vi "9217 4Ch RTD Input.vi"(1 "9217 I/O":T1={"9217 RTD0"="NI 9217/RTD0", "9217 RTD1"="NI 9217/RTD1", "9217 RTD2"="NI 9217/RTD2", "9217 RTD3"="NI 9217/RTD3"}) -> (0 "Packets":u64[](array[numeric]))   [LabVIEW 2010]
uses:
  <vilib>/eio/EIONode/EIONode.xnode
  <vilib>/rvi/eio/nirviEIOImplementation/nirviEIOImplementation.xnode
  <vilib>/rvi/eio/common/nirviEmuTemplateMethod_noerrors.vi
  <vilib>/rvi/eio/common/nirviEmuClasses.ctl
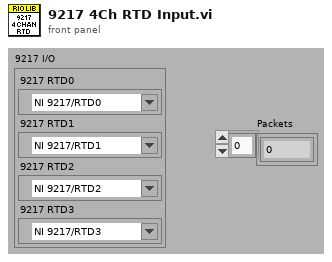
[diagram p1: front panel]
types:
  T1 = cluster{"9217 RTD0":refnum<k21>, "9217 RTD1":refnum<k21>, "9217 RTD2":refnum<k21>, "9217 RTD3":refnum<k21>}
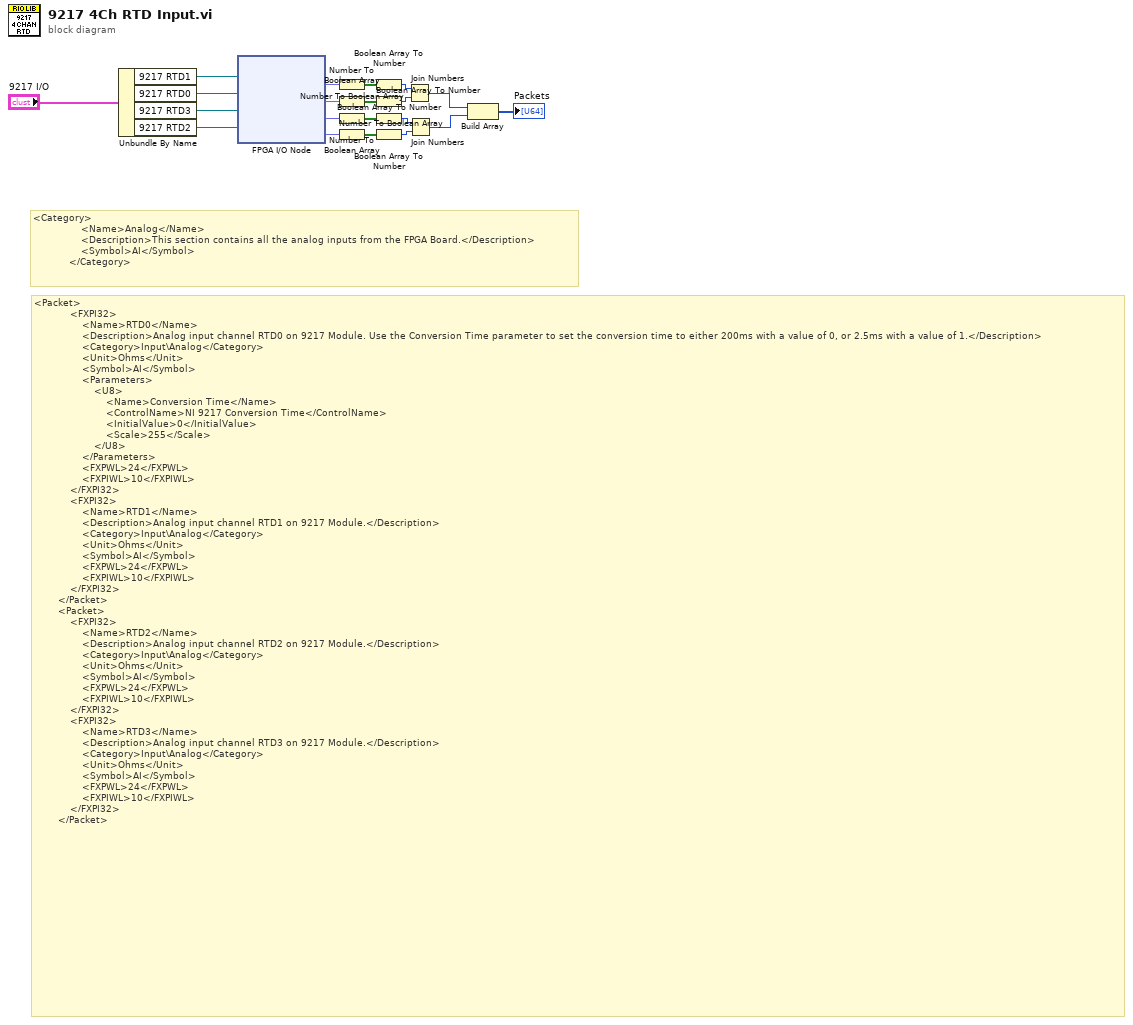
[diagram p0: block diagram]
diagram:
  # "<Category>\n                <Name>Analog</Name>\n                <Description>This section contains all the analog inputs from the FPGA Board.</Description>\n                <Symbol>AI</Symbol>\n            </Category>"
  # "<Packet>\n            <FXPI32>\n                <Name>RTD0</Name>\n                <Description>Analog input channel RTD0 on 9217 Module. Use the Conversion Time parameter to set the conversion time to either 200ms with a value of 0, or 2.5ms with a value of 1.</Description>\n                <Category>Input\\Analog</Category>\n                <Unit>Ohms</Unit>\n                <Symbol>AI</Symbol>\n                <Parameters>\n                    <U8>\n                        <Name>Conversion Time</Name>\n                        <ControlName>NI 9217 Conversion Time</ControlName>\n                        <InitialValue>0</InitialValue>\n                        <Scale>255</Scale>\n                    </U8>\n                </Parameters>\n                <FXPWL>24</FXPWL>\n                <FXPIWL>10</FXPIWL>\n            </FXPI32>\n            <FXPI32>\n                <Name>RTD1</Name>\n                <Description>Analog input channel RTD1 on 9217 Module.</Description>\n                <Category>Input\\Analog</Category>\n                <Unit>Ohms</Unit>\n                <Symbol>AI</Symbol>\n                <FXPWL>24</FXPWL>\n                <FXPIWL>10</FXPIWL>\n            </FXPI32>\n        </Packet>\n        <Packet>\n            <FXPI32>\n                <Name>RTD2</Name>\n                <Description>Analog input channel RTD2 on 9217 Module.</Description>\n                <Category>Input\\Analog</Category>\n                <Unit>Ohms</Unit>\n                <Symbol>AI</Symbol>\n                <FXPWL>24</FXPWL>\n                <FXPIWL>10</FXPIWL>\n            </FXPI32>\n            <FXPI32>\n                <Name>RTD3</Name>\n                <Description>Analog input channel RTD3 on 9217 Module.</Description>\n                <Category>Input\\Analog</Category>\n                <Unit>Ohms</Unit>\n                <Symbol>AI</Symbol>\n                <FXPWL>24</FXPWL>\n                <FXPIWL>10</FXPIWL>\n            </FXPI32>\n        </Packet>"
  n1 = Unbundle By Name("9217 I/O") -> ("9217 RTD1"=w10:refnum<k21>, "9217 RTD0"=w11:refnum<k21>, "9217 RTD3"=w12:refnum<k21>, "9217 RTD2"=w5:refnum<k21>)
  n2 = xnode "FPGA I/O Node"("FPGA I/O In"=w10, "FPGA I/O In"=w11, "FPGA I/O In"=w12, "FPGA I/O In"=w5) -> ("I/O Item"=w16:fxp<+/-,24,10>, "I/O Item"=w17:fxp<+/-,24,10>, "I/O Item"=w2:fxp<+/-,24,10>, "I/O Item"=w4:fxp<+/-,24,10>)  [unwired: 4 out]
  n3 = Number To Boolean Array(number=w16) -> (Boolean array=w13:bool[])
  n4 = Number To Boolean Array(number=w17) -> (Boolean array=w14:bool[])
  n5 = Number To Boolean Array(number=w2) -> (Boolean array=w1:bool[])
  n6 = Number To Boolean Array(number=w4) -> (Boolean array=w15:bool[])
  n7 = Boolean Array To Number(Boolean array=w13) -> (number=w18:u32)
  n8 = Boolean Array To Number(Boolean array=w14) -> (number=w19:u32)
  n9 = Boolean Array To Number(Boolean array=w1) -> (number=w3:u32)
  n10 = Boolean Array To Number(Boolean array=w15) -> (number=w20:u32)
  n11 = Join Numbers(hi=w18, lo=w19) -> ((hi.lo)=w8:u64)
  n12 = Join Numbers(hi=w3, lo=w20) -> ((hi.lo)=w9:u64)
  n13 = Build Array(w8, w9) -> (→"Packets":u64[])
